vi "Run.vi"(8 "error in (no error)":errorcluster, 11 "C37.118 PMU in":refnum<class "C37.118 PMU.lvclass">) -> (0 "error out":errorcluster, 1 "DataValid":bool, 2 "clSensorData":T1, 3 "C37.118 PMU out":refnum<class "C37.118 PMU.lvclass">)   [LabVIEW 2018, in "SensorPlugins.lvlib" / "C37.118 PMU.lvclass"]
uses:
  C37.118 PMU.lvclass
  C:/projects/ICDAS/NistPluggableModules/Sensor/SensorPlugins/SensorBaseClass/SensorBase.lvclass
  SensorShared/clSensorData.ctl
  C37.118 PMU.lvclass/C37.118 PMU.ctl
  SensorBaseClass/SensorBase.lvclass/SensorBase.ctl
  Accessors/Read DataSocket.vi
  SensorBaseClass/Accessors/Read ClkHandle.vi
  <userlib>/NIST/Socket Class/Classes/Socket.Base/Socket.Base.lvclass
  SensorShared/SensorShared.lvlib
  PmuBaseClass/PmuBase.lvclass
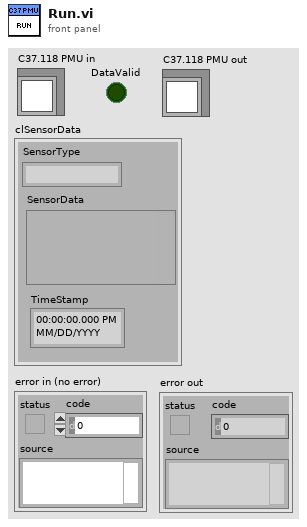
[diagram p1: front panel]
types:
  T1 = typedef "SensorShared.lvlib/clSensorData.ctl" = cluster{"SensorType":string, "SensorData":variant, "TimeStamp":timestamp}
  T2 = typedef "SensorPlugins.lvlib/PmuBase.lvclass/PMUDataType.ctl" = enum16{"undefined", "data", "header", "config 1", "config 2", "config 3", "command"}
  T3 = typedef "SensorPlugins.lvlib/PmuBase.lvclass/PmuData.ctl" = cluster{"Timestamp":dbl, "Synx":cdb[], "Freq":dbl, "ROCOF":dbl, "ID":i16}
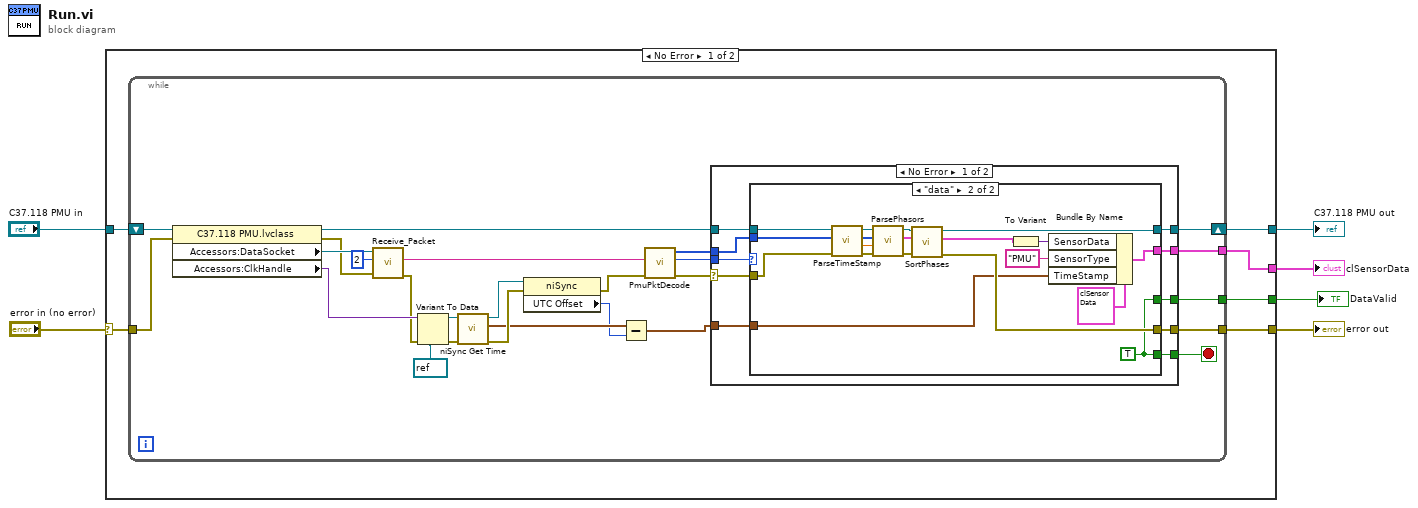
[diagram p0: block diagram]
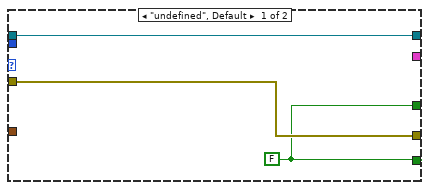
[diagram p2: hidden frame]
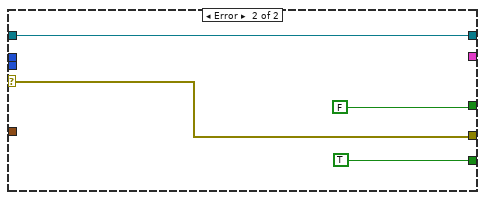
[diagram p3: hidden frame]
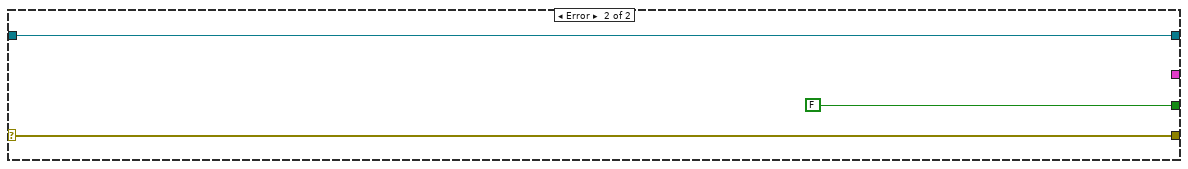
[diagram p4: hidden frame]
diagram:
  n1 = case shown="No Error" "error in (no error)" {
    selector: "error in (no error)" -> [w11 w77]
    tunnel: [w9 w77] -> w5
    tunnel: "C37.118 PMU in" -> [w12 w76]
    tunnel: [w10 w76] -> w3
    tunnel: [w8 _] -> w2
    tunnel: [w7 FALSE] -> w1
    frame No Error {
      n2 = while {
        tunnel: w11 -> [w35]
        shift-right: [w31] -> w10
        shift-left: w12 -> [w38]
        tunnel: [w29] -> w9
        tunnel: [w28] -> w8
        tunnel: [w27] -> w7
        stop <- w30 stop-if-true
        n3 = property class="C37.118 PMU.lvclass"(reference=w38, error in=w35) -> (reference out=w32:refnum<class "C37.118 PMU.lvclass">, error out=w36:errorcluster, "Accessors:DataSocket"=w37:refnum<class "Socket.Base.lvclass">, "Accessors:ClkHandle"=w26:variant)
        n4 = call-dynamic "Receive_Packet.vi"("error in (no error)"=w36, "bufsize (0)"=u32 2, "Socket.Base in"=w37) -> ("error out"=w25:errorcluster, "data_out"=w33:string)  [unwired: 5 in, 2 out]
        n5 = Variant To Data(error in=w25, type=refnum<k15> refnum ("instrument handle out"), Variant=w26) -> (data=w22:refnum<k15>, error out=w24:errorcluster)
        n6 = call <instrlib>:"niSync Get Time.vi"("error in (no error)"=w24, "instrument handle"=w22) -> ("error out"=w17:errorcluster, "time"=w16:timestamp, "instrument handle out"=w18:refnum<k15>)  [unwired: 5 in]
        n7 = property class="niSync"(reference=w18, error in=w17) -> (error out=w14:errorcluster, "UTC Offset"=w15:i32)  [unwired: 1 out]
        n8 = Subtract(x=w16, y=w15) -> (x-y=w13:timestamp)
        n9 = call "PmuPktDecode.vi"("error in (no error)"=w14, "PktData"=w33) -> ("error out"=w19:errorcluster, "PMUDataType"=w20:T2, "PktData"=w21:u8[])  [unwired: 5 in, 2 out]
        n10 = case shown="No Error" w19 {
          selector: w19 -> [w41 w72]
          tunnel: w32 -> [w48 w73]
          tunnel: [w47 w73] -> w31
          tunnel: w21 -> [w46 _]
          tunnel: w20 -> [w45 _]
          tunnel: [w44 TRUE] -> w30
          tunnel: [w43 w72] -> w29
          tunnel: [w42 _] -> w28
          tunnel: [w40 FALSE] -> w27
          tunnel: w13 -> [w39 _]
          frame No Error {
            n11 = case shown="\"data\"" w45 {
              tunnel: w48 -> [w51 w70]
              tunnel: [w51 w55] -> w47
              tunnel: w46 -> [_ w69]
              tunnel: [w49 w53] -> w44
              tunnel: w41 -> [w50 w68]
              tunnel: [w50 w56] -> w43
              tunnel: [_ w60] -> w42
              tunnel: [w49 w53] -> w40
              tunnel: w39 -> [_ w52]
              frame "undefined", Default {
                w49 = FALSE
              }
              frame "data" {
                w53 = TRUE
                n12 = call "ParseTimeStamp.vi"("error in (no error)"=w68, "PktData"=w69, "C37.118 PMU in"=w70) -> ("error out"=w67:errorcluster, "Seconds"=w64:ext, "PktData"=w65:u8[], "C37.118 PMU out"=w66:refnum<class "C37.118 PMU.lvclass">)  [unwired: 2 in, 3 out]
                n13 = call "ParsePhasors.vi"("error in (no error)"=w67, "TimeStamp"=w64, "PktData"=w65, "C37.118 PMU in"=w66) -> ("error out"=w59:errorcluster, "PmuReport"=w58:T3, "C37.118 PMU out"=w57:refnum<class "C37.118 PMU.lvclass">)  [unwired: 5 in]
                n14 = call "SortPhases.vi"("error in (no error)"=w59, "PmuReport"=w58, "C37.118 PMU in"=w57) -> ("error out"=w56:errorcluster, "PmuReport 2"=w54:T3, "C37.118 PMU out"=w55:refnum<class "C37.118 PMU.lvclass">)  [unwired: 6 in]
                n15 = To Variant(anything=w54) -> (Variant=w62:variant)
                n16 = Bundle By Name(cluster=T1 {"SensorType"="", "SensorData"=variant, "TimeStamp"=timestamp(0 s since 1904-01-01)} ("clSensorData"), "SensorData"=w62, "SensorType"="PMU", "TimeStamp"=w52) -> (w60:T1)
              }
            }
          }
          frame Error {
          }
        }
      }
    }
    frame Error {
    }
  }
  "error out" <- w5
  "C37.118 PMU out" <- w3
  "clSensorData" <- w2
  "DataValid" <- w1
